vi "Client Cancel Call Context.vi"(8 "error in":errorcluster, 11 "Call ID in":T1) -> (0 "error out":errorcluster)   [LabVIEW 2019, in "grpc-lvsupport.lvlib"]
uses:
  grpc-lvsupport.lvlib
  Shared/grpcId.ctl
  <vilib>/Utility/error.llb/Error Cluster From Error Code.vi
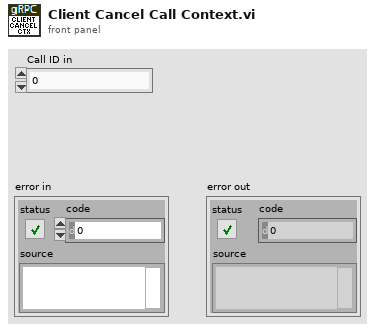
[diagram p1: front panel]
types:
  T1 = typedef "grpc-lvsupport.lvlib/grpcId.ctl" = u64
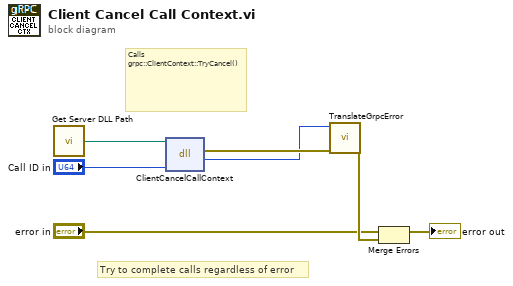
[diagram p0: block diagram]
diagram:
  # "Calls \ngrpc::ClientContext::TryCancel()"
  # "Try to complete calls regardless of error"
  n1 = call "Get Server DLL Path.vi"() -> ("Server dll path"=w5:path)
  n2 = dll-call lib="?" fn="ClientCancelCallContext"(path in=w5, "contextId"="Call ID in") -> (error out=w7:errorcluster, "return type"=w4:i32)  [unwired: 3 in, 1 out]
  n3 = call "TranslateGrpcError.vi"("error in"=w7, "Error Code"=w4) -> ("error out"=w3:errorcluster)  [unwired: 9 in]
  n4 = Merge Errors("error in", w3) -> (→"error out":errorcluster)
